vi "get Screen Dimensions.vi"(11 "Scene in":refnum<class "Scene.lvclass">) -> (3 "Rectangle Dimensions":T1)   [LabVIEW 2020, in "Scene.lvclass"]
uses:
  Scene.lvclass
  Scene.lvclass/Scene.ctl
  Graphics/Libraries/Raster/Rectangle Dimensions.ctl
  Graphics/Libraries/Raster/Raster.lvlib
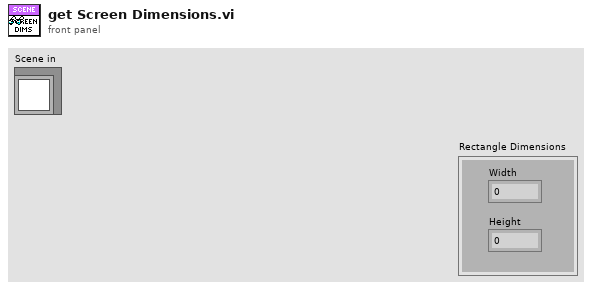
[diagram p1: front panel]
types:
  T1 = typedef "Raster.lvlib/Rectangle Dimensions.ctl" = cluster{"Width":u32, "Height":u32}
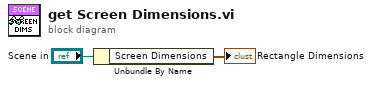
[diagram p0: block diagram]
diagram:
  n1 = Unbundle By Name("Scene in") -> ("Screen Dimensions"=→"Rectangle Dimensions":T1)
